vi "FinalReportResult_GUI.vi"(5 "TXID":string="508", 7 "RXID":string="509", 9 "BOUNCEID":string="509", 11 "error in (no error)":errorcluster, 12 "bypass git(t)":bool, 13 "Run Final Report (T)":bool=TRUE) -> (1 "standard output":string, 2 "result(ary)":string[](array[string]), 3 "pass?(t)":bool, 4 "This VI":refnum<vi>, 15 "error out":errorcluster)   [LabVIEW 2018]
panel:
  in  "stop":bool
  out "Name(str)":string
  out "Version":string
  out "tag(str)":string
  out "index of element":i32
  out "RESULT (P/F)":string
  in  "ini file(path)":path=path "C:/3500004_TetraProductionReportGenerator/testreport.ini"
  out "standard error":string
  out "DUT S/N":string
  out "git log":string="#Gitlog Commit: 0186ebcab8281aa6b5f68bf5660db075c4f76a49\n#Gitlog Author: ColinMRG <69155417+ColinMRG@users.noreply.github.com>\n#Gitlog Date:   Tue Sep 13 16:40:31 2022 -0400\n#Gitlog ComputerName: HAMPTON\r\n\r\n"
  out "GitStatus":string="C:\\3500004_TetraProductionReportGenerator\r\nIS  Up to Date with the Main HEAD\r\nIS  Up to Date with the Computer\r\n\r\n#Gitlog Commit: 0186ebcab8281aa6b5f68bf5660db075c4f76a49\n#Gitlog Author: ColinMRG <69155417+ColinMRG@users.noreply.github.com>\n#Gitlog Date:   Tue Sep 13 16:40:31 2022 -0400\n#Gitlog ComputerName: HAMPTON\r\n\r\n"
  out ".ini file(data)":string
  # "Process the result of Tetra WAM rev_C final test files"
  # "Input Data From Post Processer"
  # "Result"
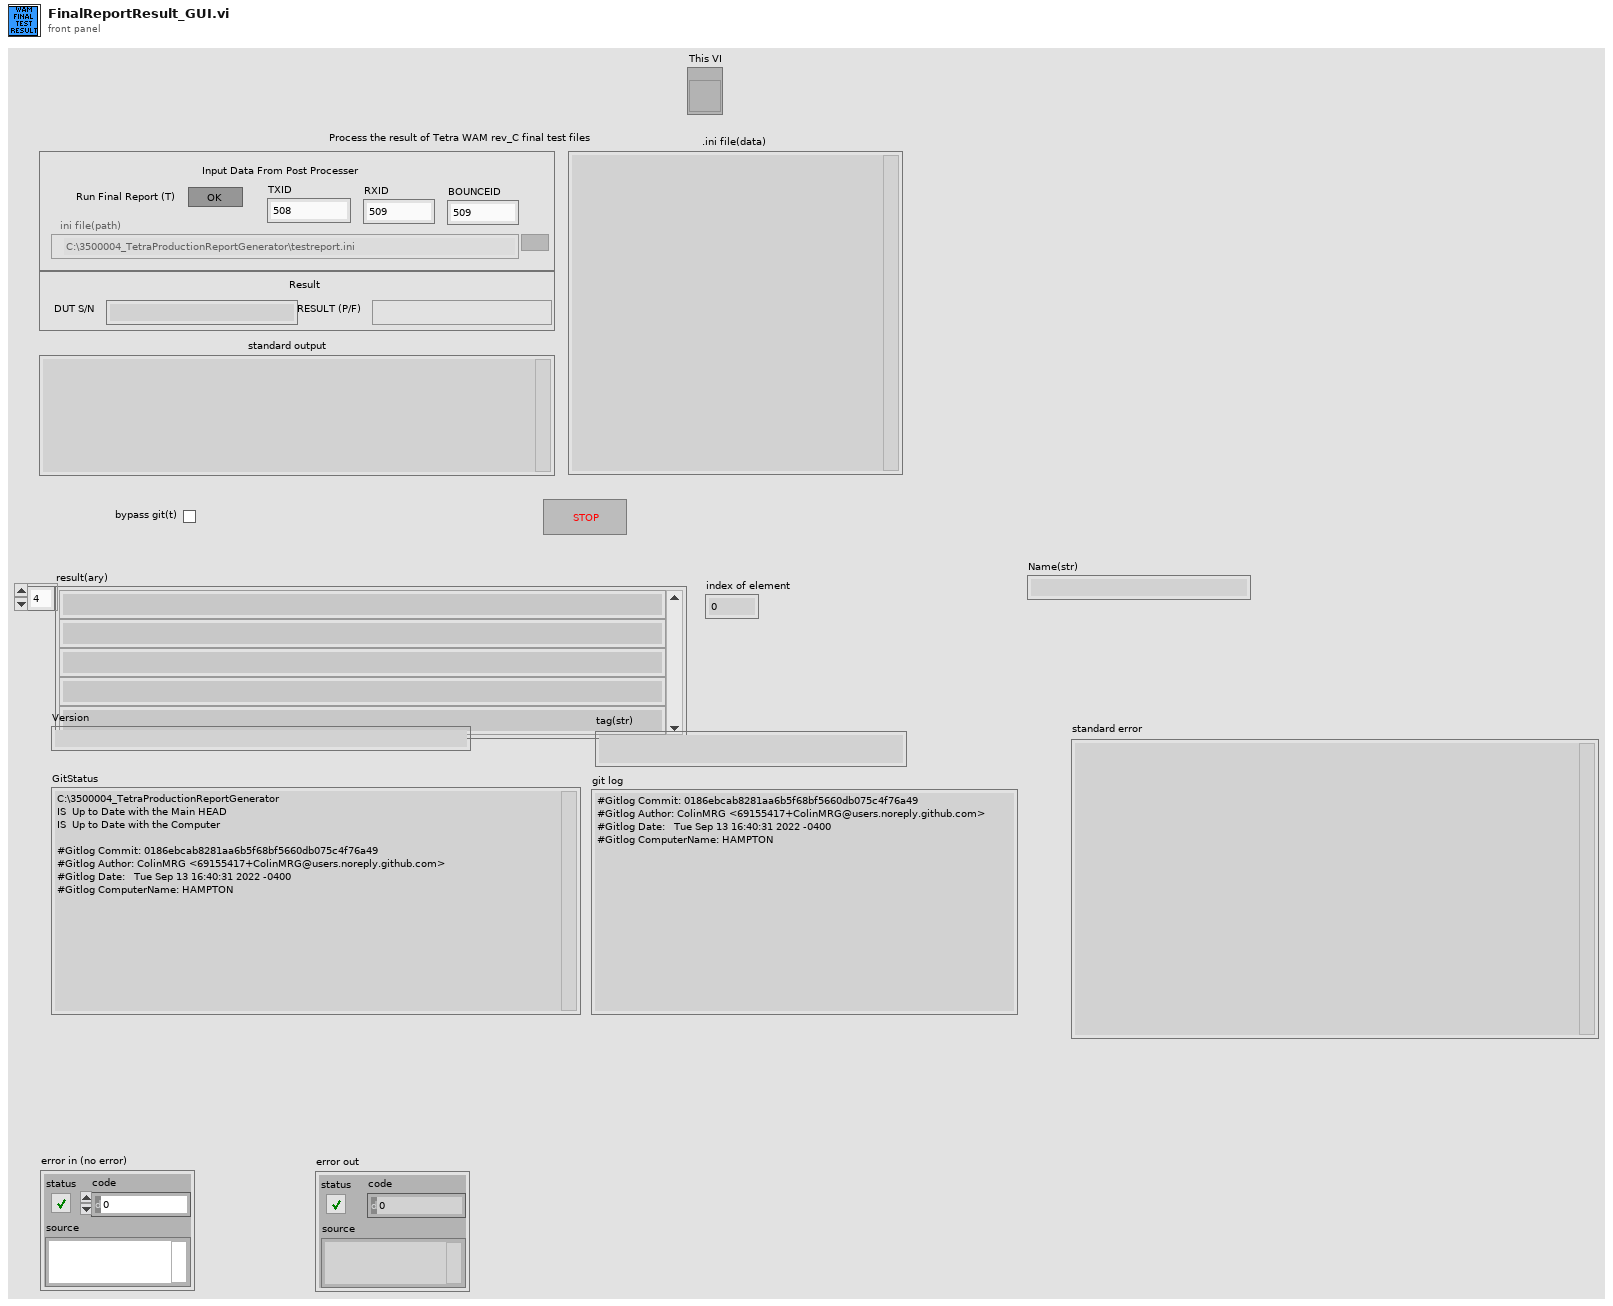
[diagram p1: front panel]
types:
  T1 = enum32{"Invalid", "Standard", "Closed", "Hidden", "Minimized", "Maximized"}
  T2 = enum16{"Left Button", "Center Button", "Right Button", "Window Close"}
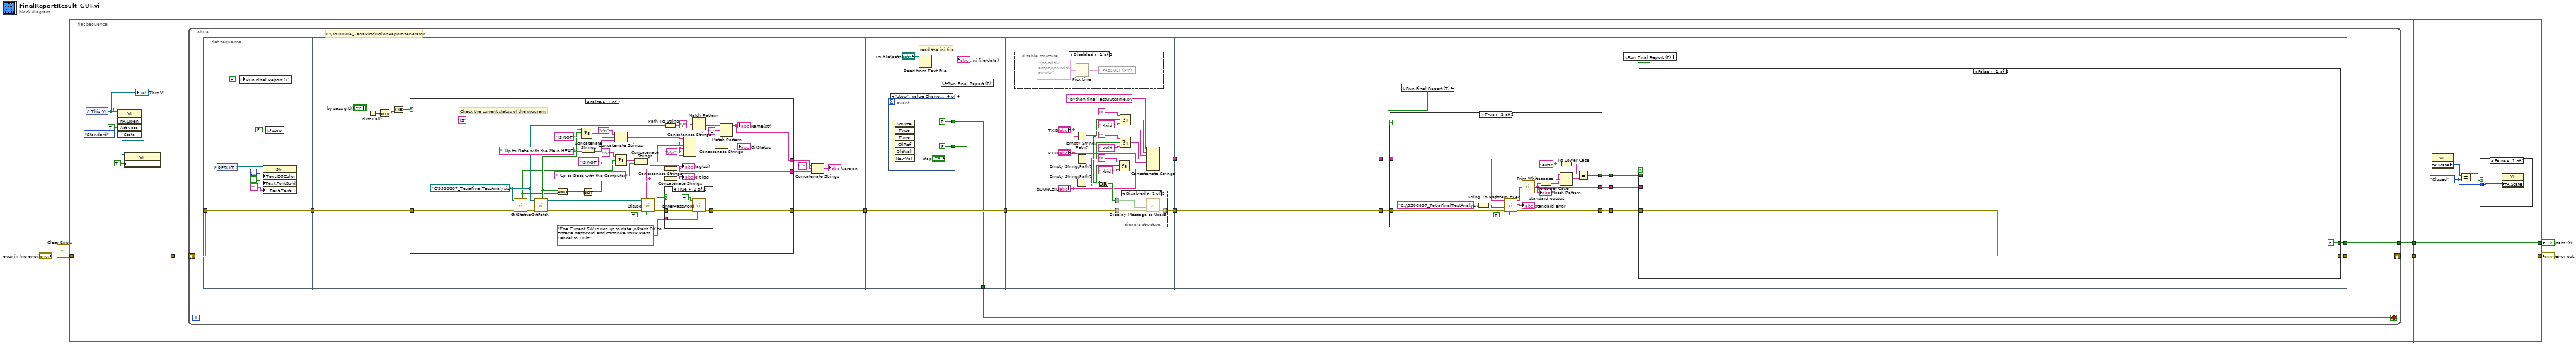
[diagram p0: block diagram]
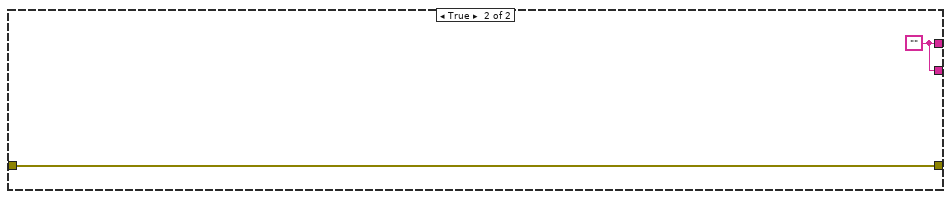
[diagram p3: hidden frame]
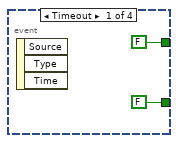
[diagram p4: hidden frame]
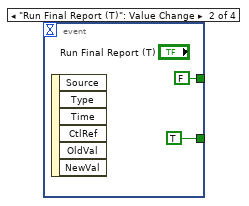
[diagram p5: hidden frame]
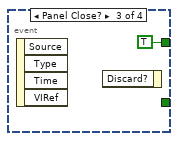
[diagram p6: hidden frame]
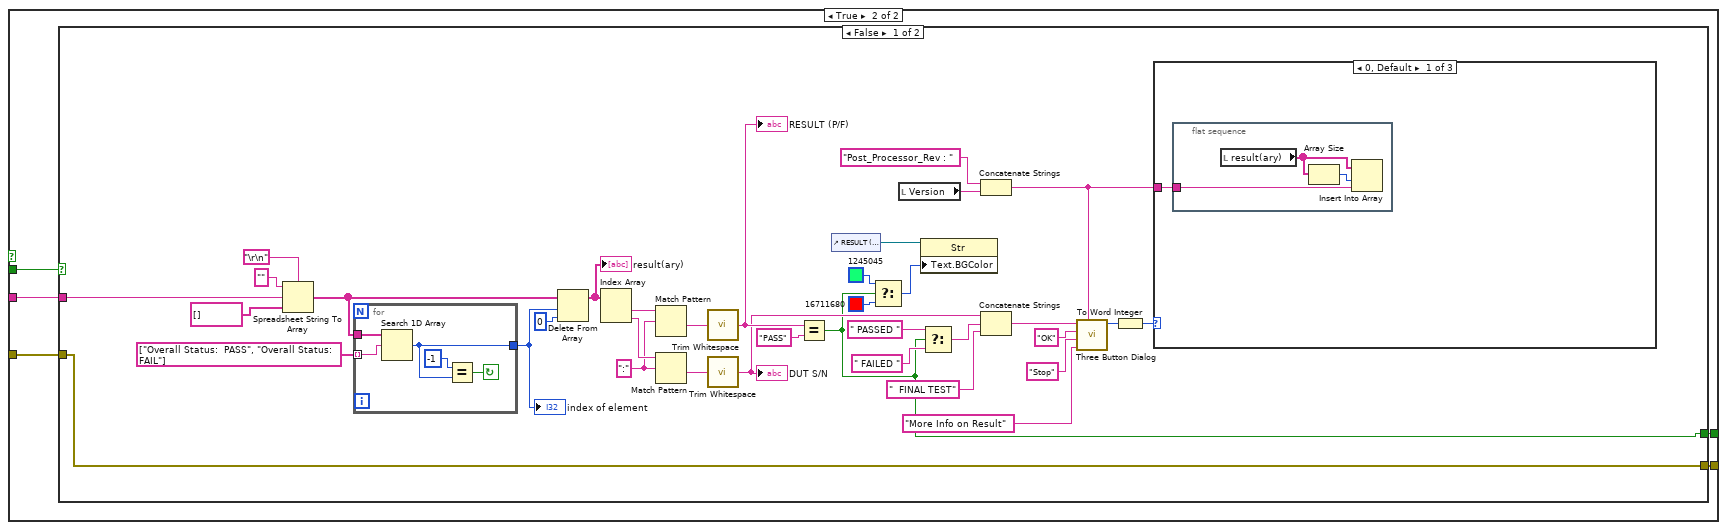
[diagram p10: hidden frame]
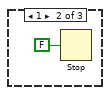
[diagram p11: hidden frame]
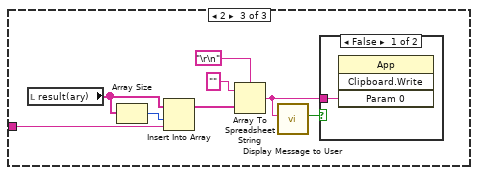
[diagram p12: hidden frame]
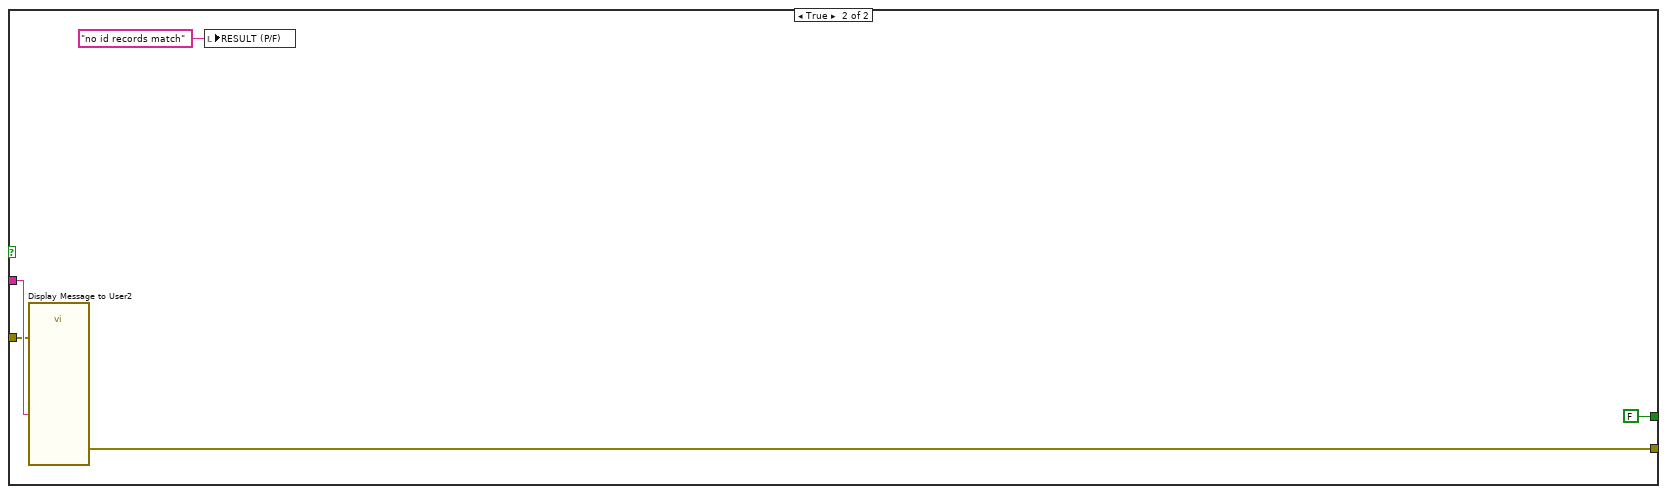
[diagram p14: hidden frame]
diagram:
  n1 = call <vilib>:"Clear Errors.vi"("error in (no error)"="error in (no error)") -> ("error out"=w5:errorcluster)  [unwired: 5 in, 1 out]
  n2 = flat-sequence {
    tunnel: w5 -> [w12]
    tunnel: [w12] -> w3
    tunnel: w3 -> [w14]
    tunnel: [w15] -> w2
    tunnel: [w13] -> w1
    tunnel: [w228] -> w4
    tunnel: [w229] -> w6
    tunnel: w2 -> [w229]
    tunnel: w1 -> [w228]
    frame #0 {
      n3 = control-ref of="This VI"() -> (w8:refnum<vi>)
      "This VI" <- w8
      n4 = invoke class="VI" method="FP.Open"(reference=w8, "Activate"=TRUE ("Activate?"), "State"=T1."Standard") -> ()  [unwired: 2 in, 5 out]
      n5 = property class="VI"(reference=w8, "Front Panel.IsFrontmost"=TRUE ("Front Panel Window:Is Frontmost")) -> ()  [unwired: 1 in, 2 out]
    }
    frame #1 {
      n6 = while {
        tunnel: [w17] -> w13
        shift-right: [w19] -> w15
        shift-left: w14 -> [w18]
        stop <- w16 stop-if-true
        # "C:\\3500004_TetraProductionReportGenerator"
        n7 = flat-sequence {
          tunnel: w18 -> [w36]
          tunnel: [w36] -> w29
          tunnel: [w45] -> w28
          tunnel: w29 -> [w46]
          tunnel: [w95] -> w27
          tunnel: w28 -> [w95]
          tunnel: [w92] -> w16
          tunnel: [w121] -> w26
          tunnel: [w116] -> w25
          tunnel: w27 -> [w117]
          tunnel: w26 -> [w130]
          tunnel: [w130] -> w24
          tunnel: w25 -> [w129]
          tunnel: [w129] -> w23
          tunnel: w24 -> [w136]
          tunnel: [w135] -> w22
          tunnel: [w133] -> w21
          tunnel: w23 -> [w134]
          tunnel: [w132] -> w20
          tunnel: w22 -> [w154]
          tunnel: w21 -> [w157]
          tunnel: [w155] -> w19
          tunnel: w20 -> [w156]
          tunnel: [w153] -> w17
          frame #0 {
            n8 = control-ref of="RESULT (P/F)"() -> (w35:refnum<vi>)
            n9 = local write "Run Final Report (T)"(FALSE ("Run Final Report (T)")) -> ()
            n10 = property class="Str"(reference=w35, "Text.BGColor"=u32 16777216, "Text.FontBold"=TRUE ("Text.Font:Bold"), "Text.Text"="") -> ()  [unwired: 1 in, 2 out]
            n11 = local write "stop"(FALSE ("stop")) -> ()
          }
          frame #1 {
            n12 = First Call?() -> (First Call?: T/F=w42:bool)
            n13 = Not(x=w42) -> (.not. x?=w41:bool)
            n14 = Or(x="bypass git(t)", y=w41) -> (x .or. y?=w43:bool)
            n15 = case shown="False" w43 {
              tunnel: w46 -> [w81 w90]
              tunnel: [w78 w90] -> w45
              tunnel: [w48 w89] -> w38
              tunnel: [w47 w89] -> w37
              frame False {
                w60 = "\r\n"
                w83 = path "C:/3500007_TetraFinalTestAnalysis" ("Directory (leave empty for relative)")
                # "Check the current status of the program"
                n16 = call "GitStatus.vi"("error in (no error)"=w81, "Directory (leave empty for relative)"=w83) -> ("error out"=w70:errorcluster, "Git Ok?(t)"=w56:bool)  [unwired: 6 in, 2 out]
                n17 = call "GitFetch.vi"("error in (no error)"=w70, "Directory (leave empty for relative)"=w83) -> ("error out"=w61:errorcluster, "directory out"=w62:path, "Git Ok?(t)"=w57:bool)  [unwired: 7 in]
                n18 = And(x=w57, y=w56) -> (x .and. y?=w49:bool)
                n19 = Select(t="IS", s=w57, f="IS NOT ") -> (s? t:f=w71:string)
                n20 = Not(x=w49) -> (.not. x?=w76:bool)
                n21 = Concatenate Strings("  Up to Date with the Main HEAD") -> (w74:string)
                n22 = Concatenate Strings("\r\n", w71, w74) -> (w65:string)
                n23 = Select(t="IS", s=w56, f="IS NOT ") -> (s? t:f=w67:string)
                n24 = Concatenate Strings(w67, "  Up to Date with the Computer") -> (w64:string)
                n25 = call "GitLog.vi"("GetCurrentTag(T)"=TRUE, "error in (no error)"=w61, "Directory (leave empty for relative)"=w62) -> ("error out"=w77:errorcluster, "git log"=w59:string, "tag"=w55:string)  [unwired: 5 in, 1 out]
                n26 = Path To String(path=w83) -> (string=w53:string)
                n27 = Concatenate Strings(w55) -> (w47:string)
                "tag(str)" <- w47
                n28 = Concatenate Strings(w59) -> (→"git log":string)
                n29 = case shown="True" w76 {
                  tunnel: "The Current SW is not up to date.\nPress OK to Enter a password and continue \nOR Press Cancel to Quit" ("Message") -> [_ w88]
                  tunnel: [w84 w87] -> w78
                  tunnel: w77 -> [w84 w86]
                  frame False {
                  }
                  frame True {
                    n30 = call "EnterPassword.vi"("Message"=w88, "error in (no error)"=w86, "Enable(t)"=TRUE) -> ("error out"=w87:errorcluster)  [unwired: 6 in, 2 out]
                  }
                }
                n31 = Concatenate Strings(w65, w60, w64, w60, w60, w59) -> (w58:string)
                n32 = Match Pattern(string=w53, regular expression="\\") -> (after substring=w51:string)  [unwired: 1 in, 3 out]
                n33 = Concatenate Strings(w58) -> (→"GitStatus":string)
                n34 = Match Pattern(string=w51, regular expression="_") -> (before substring=w48:string)  [unwired: 1 in, 3 out]
                "Name(str)" <- w48
              }
              frame True {
                w89 = ""
              }
            }
            n35 = Concatenate Strings(w38, "  " ("string"), w37) -> (→"Version":string)
          }
          frame #2 {
            # "read the ini file"
            n36 = event shown="[3] \"stop\": Value Change" {
              selector: _ -> [_ _ _ _]
              dyn-events: _ -> [_ _ _ _]
              timeout: _ -> [_ _ _ _]
              tunnel: [FALSE FALSE TRUE TRUE] -> w92
              tunnel: [FALSE ("Run Final Report (T)") TRUE ("Run Final Report (T)") _ FALSE ("Run Final Report (T)")] -> w91
              event Timeout {
                n37 = event-data() -> ()  [unwired: 1 in, 3 out]
              }
              event "Run Final Report (T)": Value Change {
                n38 = event-data() -> ()  [unwired: 1 in, 6 out]
              }
              event Panel Close? {
                n39 = event-data() -> ()  [unwired: 1 in, 4 out]
                n40 = event-data() -> ()  [unwired: 2 in, 1 out]
              }
              event "stop": Value Change {
                n41 = event-data() -> ()  [unwired: 1 in, 6 out]
              }
            }
            n42 = Read from Text File(file (use dialog)="ini file(path)") -> (text=→".ini file(data)":string)  [unwired: 3 in, 3 out]
            n43 = local write "Run Final Report (T)"(w91) -> ()
          }
          frame #3 {
            n44 = disable-structure shown="Disabled" {
              frame Disabled {
                n45 = Pick Line(multi-line string="\n<txid> empty\n<rxid> empty") -> (output string=w123:string)  [unwired: 2 in]
                n46 = local write "RESULT (P/F)"(w123) -> ()
              }
              frame Enabled {
              }
            }
            n47 = Empty String/Path?(string/path="BOUNCEID") -> (empty?=w111:bool)
            n48 = Empty String/Path?(string/path="TXID") -> (empty?=w105:bool)
            n49 = Empty String/Path?(string/path="RXID") -> (empty?=w109:bool)
            n50 = Or(x=w105, y=w109) -> (x .or. y?=w118:bool)
            n51 = disable-structure shown="Disabled" {
              disable-tunnel: w118 -> [w127 _]
              disable-tunnel: w117 -> [w126 w128]
              disable-tunnel: [w125 w128] -> w116
              frame Disabled {
                n52 = call "Display Message to User3"("error in (no error)"=w126, "Enable"=w127) -> ("error out"=w125:errorcluster)  [unwired: 8 in, 1 out]
              }
              frame Enabled {
              }
            }
            n53 = Select(t="", s=w111, f=" -bid " ("string")) -> (s? t:f=w113:string)
            n54 = Select(t="", s=w105, f=" -txid " ("string")) -> (s? t:f=w106:string)
            n55 = Select(t="", s=w109, f=" -rxid " ("string")) -> (s? t:f=w108:string)
            n56 = Concatenate Strings("python finalTestOutcome.py" ("command line"), w106, "TXID", w108, "RXID", w113, "BOUNCEID") -> (w121:string)
          }
          frame #4 {
          }
          frame #5 {
            n57 = local read "Run Final Report (T)"() -> (w131:bool)
            n58 = case shown="True" w131 {
              tunnel: w136 -> [_ w150]
              tunnel: [w137 w149] -> w135
              tunnel: w134 -> [w137 w147]
              tunnel: [_ w145] -> w133
              tunnel: [_ w138] -> w132
              frame False {
              }
              frame True {
                w143 = "error" ("regular expression")
                n59 = String To Path(string="C:\\3500007_TetraFinalTestAnalysis") -> (path=w140:path)
                n60 = call <vilib>:"System Exec.vi"("run minimized? (F)"=TRUE, "error in (no error)"=w147, "working directory"=w140, "command line"=w150) -> ("error out"=w149:errorcluster, "standard error"=→"standard error":string, "standard output"=w148:string)  [unwired: 4 in, 1 out]
                n61 = call <vilib>:"Trim Whitespace.vi"("string"=w148) -> ("trimmed string"=w145:string)  [unwired: 1 in]
                "standard output" <- w145
                n62 = To Lower Case(string=w145) -> (all lower case string=w141:string)
                n63 = To Lower Case(string=w143) -> (all lower case string=w142:string)
                n64 = Match Pattern(string=w141, regular expression=w143) -> (match substring=w144:string)  [unwired: 1 in, 3 out]
                n65 = Equal?(x=w142, y=w144) -> (x = y?=w138:bool)
              }
            }
          }
          frame #6 {
            n66 = local read "Run Final Report (T)"() -> (w152:bool)
            n67 = case shown="False" w152 {
              tunnel: w157 -> [_ w164]
              tunnel: w156 -> [_ w163]
              tunnel: [w158 w162] -> w155
              tunnel: w154 -> [w158 w161]
              tunnel: [FALSE w160] -> w153
              frame False {
              }
              frame True {
                n68 = case shown="False" w163 {
                  tunnel: w164 -> [w197 w224]
                  tunnel: [w172 w222] -> w162
                  tunnel: w161 -> [w172 w221]
                  tunnel: [w180 FALSE] -> w160
                  frame False {
                    w193 = ":" ("regular expression")
                    n69 = Spreadsheet String To Array(delimiter (Tab)="\r\n", format string="", spreadsheet string=w197, array type (2D Dbl)=string[] []) -> (array=w171:string[])
                    n70 = for {
                      tunnel: w171 -> [w205]
                      tunnel: string[] ["Overall Status:  PASS", "Overall Status:  FAIL"] ("array type (2D Dbl)") -> [w204] mode=indexing
                      tunnel: [w203] -> w170
                      stop <- w201 continue-if-true
                      n71 = Search 1D Array(1D array=w205, element=w204) -> (index of element=w203:i32)  [unwired: 1 in]
                      n72 = Equal?(x=-1, y=w203) -> (x = y?=w201:bool)
                    }
                    "index of element" <- w170
                    n73 = Delete From Array(array=w171, length=w170, index=0) -> (array with subset deleted=w169:string[])  [unwired: 1 out]
                    "result(ary)" <- w169
                    n74 = Index Array(array=w169) -> (element #1=w195:string, element #2=w194:string)  [unwired: 2 in]
                    n75 = Match Pattern(string=w195, regular expression=w193) -> (after substring=w191:string)  [unwired: 1 in, 3 out]
                    n76 = Match Pattern(string=w194, regular expression=w193) -> (after substring=w192:string)  [unwired: 1 in, 3 out]
                    n77 = call <vilib>:"Trim Whitespace.vi"("string"=w191) -> ("trimmed string"=w190:string)  [unwired: 1 in]
                    "RESULT (P/F)" <- w190
                    n78 = call <vilib>:"Trim Whitespace.vi"("string"=w192) -> ("trimmed string"=w188:string)  [unwired: 1 in]
                    "DUT S/N" <- w188
                    n79 = Equal?(x=w190, y="PASS") -> (x = y?=w180:bool)
                    n80 = control-ref of="RESULT (P/F)"() -> (w182:refnum<vi>)
                    n81 = Select(t=u32 1245045, s=w180, f=u32 16711680) -> (s? t:f=w183:u32)
                    n82 = local read "Version"() -> (w168:string)
                    n83 = property class="Str"(reference=w182, "Text.BGColor"=w183) -> ()  [unwired: 1 in, 2 out]
                    n84 = Select(t=" PASSED " ("y"), s=w180, f=" FAILED " ("y")) -> (s? t:f=w186:string)
                    n85 = Concatenate Strings("Post_Processor_Rev : " ("string"), w168) -> (w167:string)
                    n86 = Concatenate Strings(w188, w186, "  FINAL TEST" ("string")) -> (w178:string)
                    n87 = call <vilib>:"Three Button Dialog.vi"("Window Title (\"\")"=w167, "Right Button Text (\"Cancel\")"="More Info on Result" ("Right Button Text (\"Cancel\")"), "Center Button Text (\"No\")"="Stop" ("Center Button Text (\"No\")"), "Left Button Text (\"Yes\")"="OK" ("Left Button Text (\"Yes\")"), "message"=w178) -> ("Which Button?"=w174:T2)  [unwired: 6 in]
                    n88 = To Word Integer(number=w174) -> (16bit integer=w173:i16)
                    n89 = case shown="0, Default" w173 {
                      tunnel: w167 -> [w206 _ w213]
                      frame 0, Default {
                        n90 = flat-sequence {
                          tunnel: w206 -> [w208]
                          frame #0 {
                            n91 = local read "result(ary)"() -> (w209:string[])
                            n92 = Array Size(array=w209) -> (size(s)=w207:i32)
                            n93 = Insert Into Array(array=w209, index=w207, new element=w208) -> ()  [unwired: 1 out]
                          }
                        }
                      }
                      frame 1 {
                        n94 = Stop(stop? (T)=FALSE) -> ()
                      }
                      frame 2 {
                        n95 = local read "result(ary)"() -> (w214:string[])
                        n96 = Array Size(array=w214) -> (size(s)=w212:i32)
                        n97 = Insert Into Array(array=w214, index=w212, new element=w213) -> (w211:string[])
                        n98 = Array To Spreadsheet String(delimiter (Tab)="\r\n", array=w211, 3:"" ("format string")) -> (spreadsheet string=w217:string)
                        n99 = call "Display Message to User"("Message"=w217) -> ("OK"=w218:bool)  [unwired: 9 in, 1 out]
                        n100 = case shown="False" w218 {
                          tunnel: w217 -> [w219 _]
                          frame False {
                            n101 = invoke class="App" method="Clipboard.Write"("Param 0"=w219) -> ()  [unwired: 3 in, 4 out]
                          }
                          frame True {
                          }
                        }
                      }
                    }
                  }
                  frame True {
                    n102 = call "Display Message to User2"("error in (no error)"=w221, "Message"=w224) -> ("error out"=w222:errorcluster)  [unwired: 8 in, 1 out]
                    n103 = local write "RESULT (P/F)"("no id records match" ("RESULT (P/F)")) -> ()
                  }
                }
              }
            }
          }
        }
      }
    }
    frame #2 {
      w225 = T1."Closed" ("y")
      n104 = property class="VI"() -> ("FP.State"=w226:T1)  [unwired: 2 in, 2 out]
      n105 = Equal?(x=w226, y=w225) -> (x = y?=w227:bool)
      n106 = case shown="False" w227 {
        tunnel: w225 -> [w230 _]
        frame False {
          n107 = property class="VI"("FP.State"=w230) -> ()  [unwired: 2 in, 2 out]
        }
        frame True {
        }
      }
    }
  }
  "error out" <- w6
  "pass?(t)" <- w4
